vi "Omega Trapezoid.vi"(6 "dt":dbl, 7 "ttot":dbl, 10 "a":dbl, 11 "g":dbl) -> (2 "Thetas":dbl[](array[numeric]), 3 "Omegas":dbl[](array[numeric]))   [LabVIEW 2025]
panel:
  out "Velocity Graph":cluster{"v_rec":dbl[], "a_rec":dbl[]}[](graph)
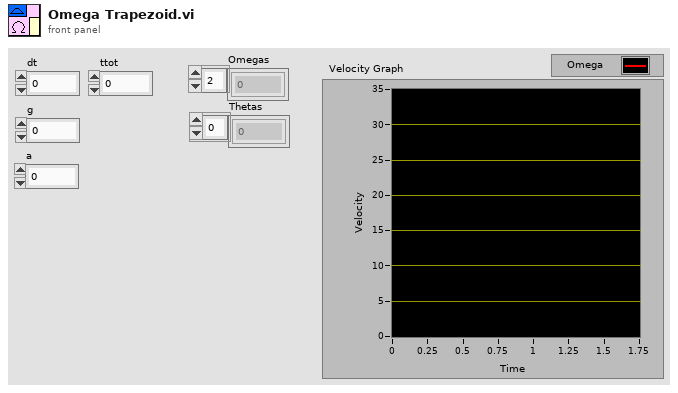
[diagram p1: front panel]
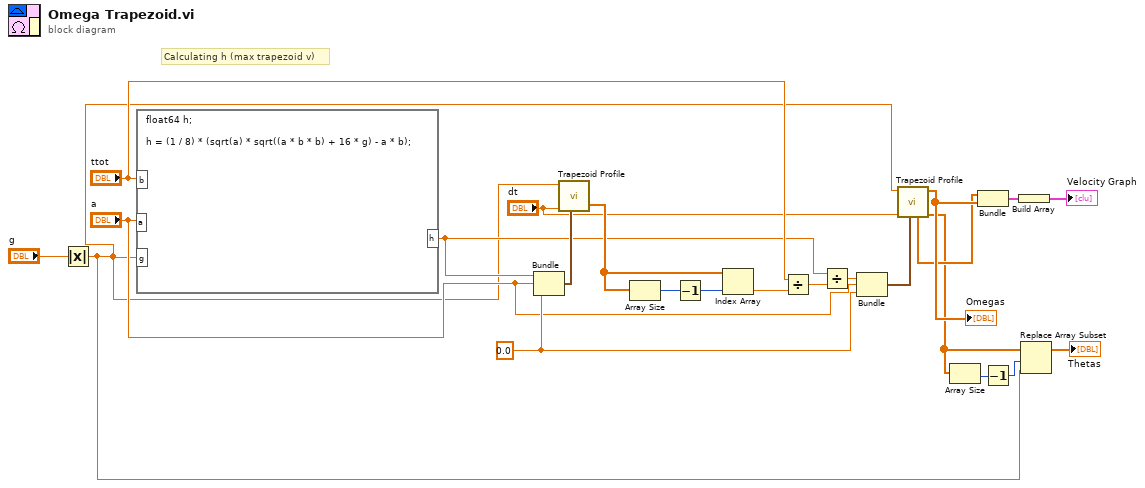
[diagram p0: block diagram]
diagram:
  w13 = 0.0 ("a")
  # "Calculating h (max trapezoid v)"
  n1 = Absolute Value(x="g") -> (abs(x)=w2:dbl)
  n2 = formula code="float64 h;\n\nh = (1 / 8) * (sqrt(a) * sqrt((a * b * b) + 16 * g) - a * b);"("a"="a", "g"=w2, "b"="ttot") -> ("h"=w16:dbl)
  n3 = Bundle(w16, "a"="a", "a"=w13) -> (w23:cluster{dbl, "a":dbl, "a":dbl})  [unwired: 1 in]
  n4 = call "Trapezoid Profile.vi"("Limits"=w23, "dt"="dt", "goal"=w2) -> ("t_rec"=w20:dbl[])  [unwired: 6 in, 2 out]
  n5 = Array Size(array=w20) -> (size(s)=w22:i32)
  n6 = Decrement(x=w22) -> (x-1=w21:i32)
  n7 = Index Array(array=w20, index=w21) -> (element=w19:dbl)
  n8 = Divide(x="ttot", y=w19) -> (x/y=w17:dbl)
  n9 = Divide(x=w16, y=w17) -> (x/y=w14:dbl)
  n10 = Bundle(w14, "a"="a", "a"=w13) -> (w11:cluster{dbl, "a":dbl, "a":dbl})  [unwired: 1 in]
  n11 = call "Trapezoid Profile.vi"("Limits"=w11, "dt"="dt", "goal"=w2) -> ("x_rec"=w5:dbl[], "v_rec"=w9:dbl[], "t_rec"=w8:dbl[])  [unwired: 6 in]
  "Omegas" <- w9
  n12 = Array Size(array=w5) -> (size(s)=w4:i32)
  n13 = Bundle("t_rec"=w8, "v_rec"=w9) -> (w7:cluster{"t_rec":dbl[], "v_rec":dbl[]})  [unwired: 1 in]
  n14 = Decrement(x=w4) -> (x-1=w3:i32)
  n15 = Build Array(w7) -> (→"Velocity Graph":cluster{"t_rec":dbl[], "v_rec":dbl[]}[])
  n16 = Replace Array Subset(array=w5, new element=w2, index=w3) -> (→"Thetas":dbl[])
